vi "Write Parent Menu.vi"(8 "error in (no error)":errorcluster, 10 "Parent Menu":string, 11 "NIVS_CD Template in":refnum<class "NIVS_CD Template.lvclass">) -> (0 "error out":errorcluster, 3 "NIVS_CD Template out":refnum<class "NIVS_CD Template.lvclass">)   [LabVIEW 2016, in "NIVS_CD Template.lvclass"]
uses:
  NIVS_CD Template.lvclass
  NIVS_CD Template.lvclass/NIVS_CD Template.ctl
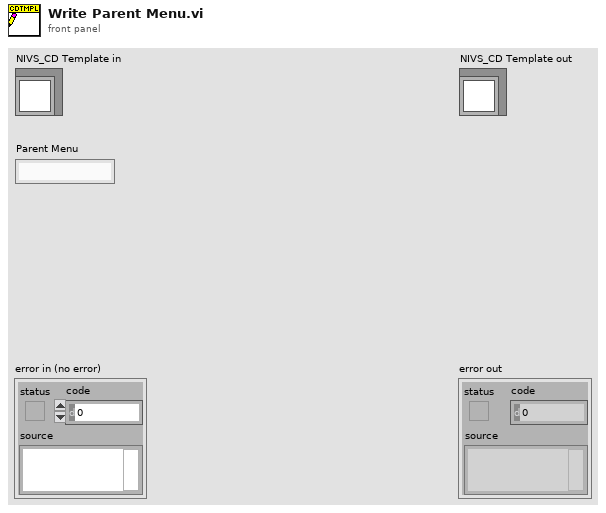
[diagram p1: front panel]
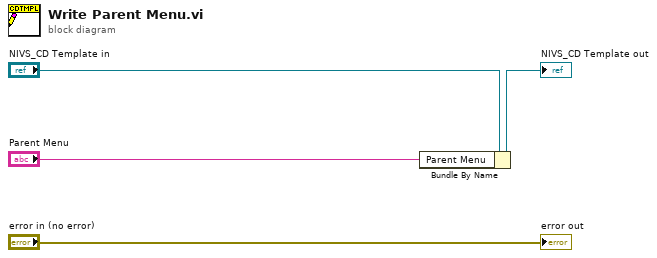
[diagram p0: block diagram]
diagram:
  n1 = Bundle By Name(cluster="NIVS_CD Template in", "Parent Menu"="Parent Menu") -> (→"NIVS_CD Template out":refnum<class "NIVS_CD Template.lvclass">)
  "error out" <- "error in (no error)"
